vi "Prepare LV to Use Icon Editor Source.vi"   [LabVIEW 2021]
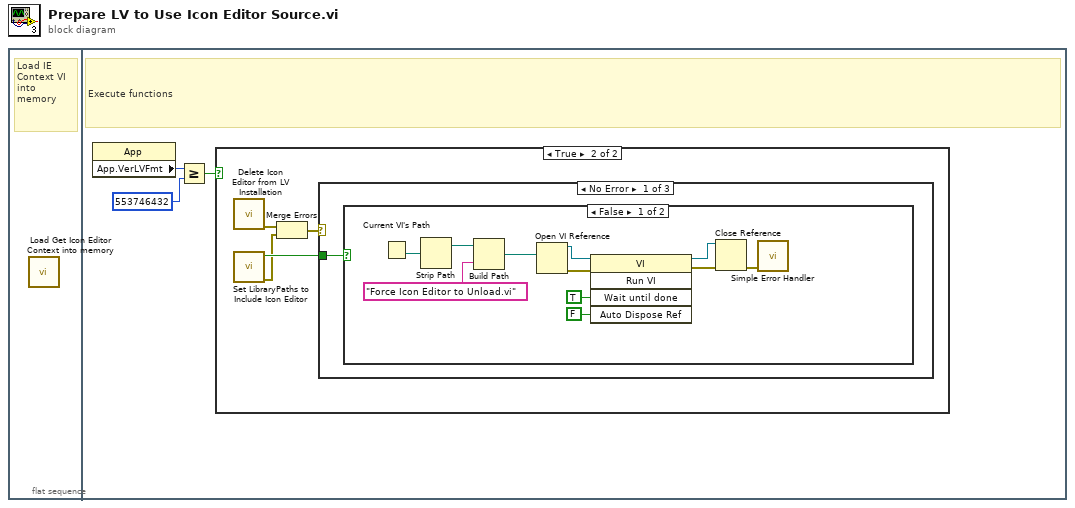
[diagram p0: block diagram]
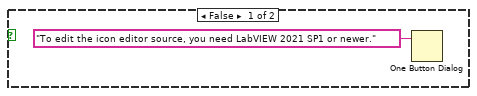
[diagram p2: hidden frame]
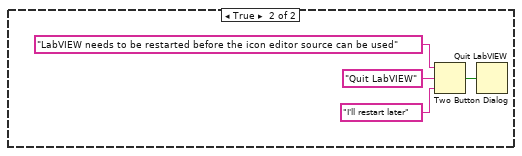
[diagram p3: hidden frame]
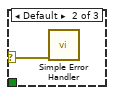
[diagram p4: hidden frame]
diagram:
  n1 = flat-sequence {
    frame #0 {
      # "Load IE Context VI into memory"
      n2 = call "Load Get Icon Editor Context into memory.vi"() -> ()  [unwired: 12 in]
    }
    frame #1 {
      # "Execute functions"
      n3 = property class="App"() -> ("App.VerLVFmt"=w3:i32)  [unwired: 2 in, 2 out]
      n4 = Greater Or Equal?(x=w3, y=553746432 ("Application:Version As Integer")) -> (x >= y?=w1:bool)
      n5 = case shown="True" w1 {
        frame False {
          n6 = One Button Dialog(message="To edit the icon editor source, you need LabVIEW 2021 SP1 or newer.") -> ()  [unwired: 1 in, 1 out]
        }
        frame True {
          n7 = call "Delete Icon Editor from LV Installation.vi"() -> ("error out"=w7:errorcluster)  [unwired: 10 in, 1 out]
          n8 = call "Set LibraryPaths to Include Icon Editor.vi"() -> ("error out"=w5:errorcluster, "config modified?"=w8:bool)  [unwired: 10 in]
          n9 = Merge Errors(w7, w5) -> (w6:errorcluster)
          n10 = case shown="No Error" w6 {
            selector: w6 -> [_ w25 _]
            tunnel: w8 -> [w9 _ _]
            frame No Error {
              n11 = case shown="False" w9 {
                frame False {
                  n12 = Current VI's Path() -> (path=w20:path)
                  n13 = Strip Path(path=w20) -> (stripped path=w19:path)  [unwired: 1 out]
                  n14 = Build Path(base path=w19, name or relative path="Force Icon Editor to Unload.vi") -> (appended path=w17:path)
                  n15 = Open VI Reference(vi path=w17) -> (vi reference=w16:refnum<vi>, error out=w15:errorcluster)  [unwired: 5 in]
                  n16 = invoke class="VI" method="Run VI"(reference=w16, error in=w15, "Wait until done"=TRUE ("Wait Until Done"), "Auto Dispose Ref"=FALSE ("Auto Dispose Reference")) -> (reference out=w11:refnum<vi>, error out=w14:errorcluster)  [unwired: 1 in, 3 out]
                  n17 = Close Reference(reference=w11, error in (no error)=w14) -> (error out=w10:errorcluster)
                  n18 = call <vilib>:"Simple Error Handler.vi"("error in (no error)"=w10) -> ()  [unwired: 4 in, 5 out]
                }
                frame True {
                  n19 = Two Button Dialog(message="LabVIEW needs to be restarted before the icon editor source can be used", 1:"I'll restart later" ("F button name (\"Cancel\")"), 2:"Quit LabVIEW" ("T button name (\"OK\")")) -> (T button?=w24:bool)
                  n20 = Quit LabVIEW(quit? (T)=w24) -> ()
                }
              }
            }
            frame Default {
              n21 = call <vilib>:"Simple Error Handler.vi"("error in (no error)"=w25) -> ()  [unwired: 4 in, 5 out]
            }
            frame Error {
              # "User cancelled, no further interaction needed"
            }
          }
        }
      }
    }
  }
